vi "DestroySelfReference.vi"(8 "error in (no error)":errorcluster, 11 "DB2":refnum<class "DB2.lvclass">) -> (0 "error out":errorcluster, 3 "DB2 out":refnum<class "DB2.lvclass">)   [LabVIEW 2022 SP3, in "DB2.lvclass"]
uses:
  DB2.lvclass
  DB2.lvclass/DB2.ctl
  <vilib>/JKI/JKI SMO/SMO/SMO.lvclass
panel:
  # "For instructions on how to use the JKI State Machine Objects, examples and video tutorials, visit:\nhttp://jki.net/state-machine-objects/\n\nJKI State Machine Objects™\nhttp://jki.net/state-machine-objects/\nCopyright (C) 2005-2015, JKI <info@jki.net>\nALL RIGHTS RESERVED"
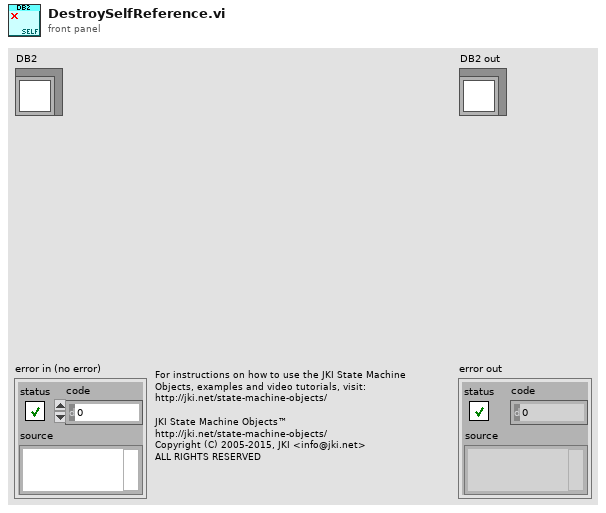
[diagram p1: front panel]
types:
  T1 = typedef "DB2.lvclass/PrivateData--Ref.ctl" = refnum<data-value>
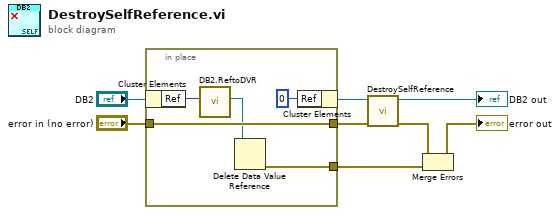
[diagram p0: block diagram]
diagram:
  n1 = in-place {
    in-place-border: [w12] -> w3
    in-place-border: "error in (no error)" -> [w11]
    in-place-border: [w11] -> w1
    n2 = in-place-cluster #1("DB2") -> ("Ref"=w10:u32)
    n3 = call "DB2.ReftoDVR.vi"("Ref"=w10) -> ("Ref"=w9:T1)  [unwired: 10 in]
    n4 = Delete Data Value Reference(data value reference=w9) -> (error out=w12:errorcluster)  [unwired: 1 in, 1 out]
    n5 = in-place-cluster #1("Ref"=u32 0) -> (w4:refnum<class "DB2.lvclass">)
  }
  n6 = call-parent "DestroySelfReference.vi"("error in (no error)"=w1, "SMO"=w4) -> ("error out"=w7:errorcluster, "SMO out"=→"DB2 out":refnum<class "DB2.lvclass">)  [unwired: 8 in]
  n7 = Merge Errors(w7, w3) -> (→"error out":errorcluster)
